vi "readMotorPodConfig.vi"(7 "Input Pod Clustor":T1, 8 "Pod Number":i32, 9 "Refnum in":T2) -> (1 "Pod Output":T1)   [LabVIEW 2014]
uses:
  <vilib>/Utility/config.llb/Config Data RefNum.ctl
  read/readI32.vi
  read/readDoubleKey.vi
  read/readBooleanKey.vi
  read/readStringKey.vi
  <vilib>/Utility/config.llb/NI_LVConfig.lvlib
panel:
  in  "error in (no error)":errorcluster
  out "Refnum out":T2
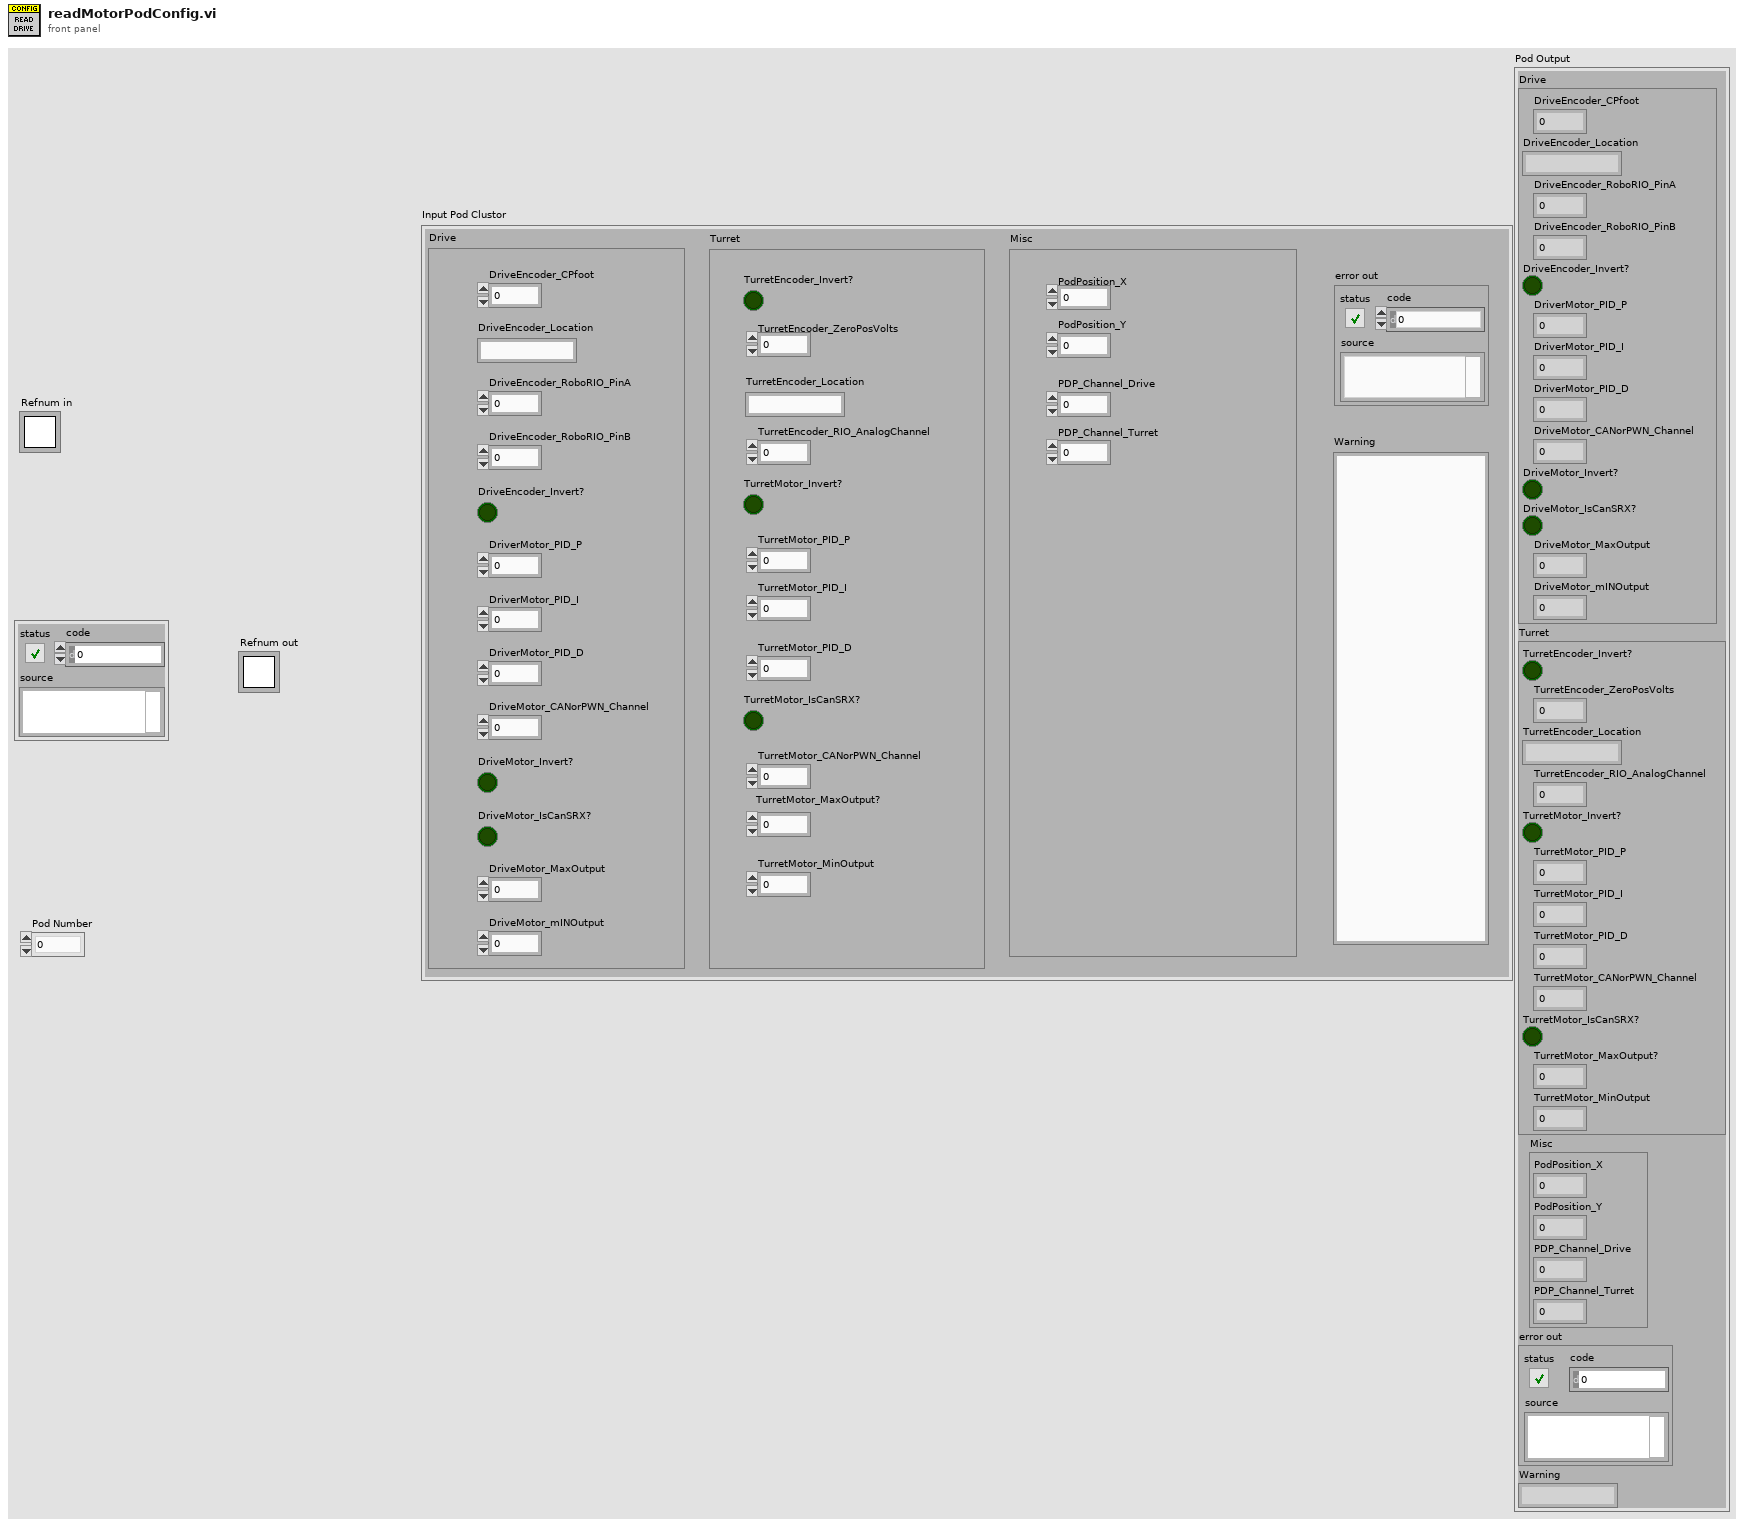
[diagram p1: front panel]
types:
  T1 = cluster{"Drive":cluster{"DriveEncoder_CPfoot":dbl, "DriveEncoder_Location":string, "DriveEncoder_RoboRIO_PinA":i32, "DriveEncoder_RoboRIO_PinB":i32, "DriveEncoder_Invert?":bool, "DriverMotor_PID_P":dbl, "DriverMotor_PID_I":dbl, "DriverMotor_PID_D":dbl, "DriveMotor_CANorPWN_Channel":i32, "DriveMotor_Invert?":bool, "DriveMotor_IsCanSRX?":bool, "DriveMotor_MaxOutput":dbl, "DriveMotor_mINOutput":dbl}, "Turret":cluster{"TurretEncoder_Invert?":bool, "TurretEncoder_ZeroPosVolts":dbl, "TurretEncoder_Location":string, "TurretEncoder_RIO_AnalogChannel":dbl, "TurretMotor_Invert?":bool, "TurretMotor_PID_P":dbl, "TurretMotor_PID_I":dbl, "TurretMotor_PID_D":dbl, "TurretMotor_CANorPWN_Channel":dbl, "TurretMotor_IsCanSRX?":bool, "TurretMotor_MaxOutput?":dbl, "TurretMotor_MinOutput":dbl}, "Misc":cluster{"PodPosition_X":dbl, "PodPosition_Y":dbl, "PDP_Channel_Drive":i32, "PDP_Channel_Turret":i32}, "error out":errorcluster, "Warning":string}
  T2 = typedef "NI_LVConfig.lvlib/Config Data RefNum.ctl" = refnum<k1>
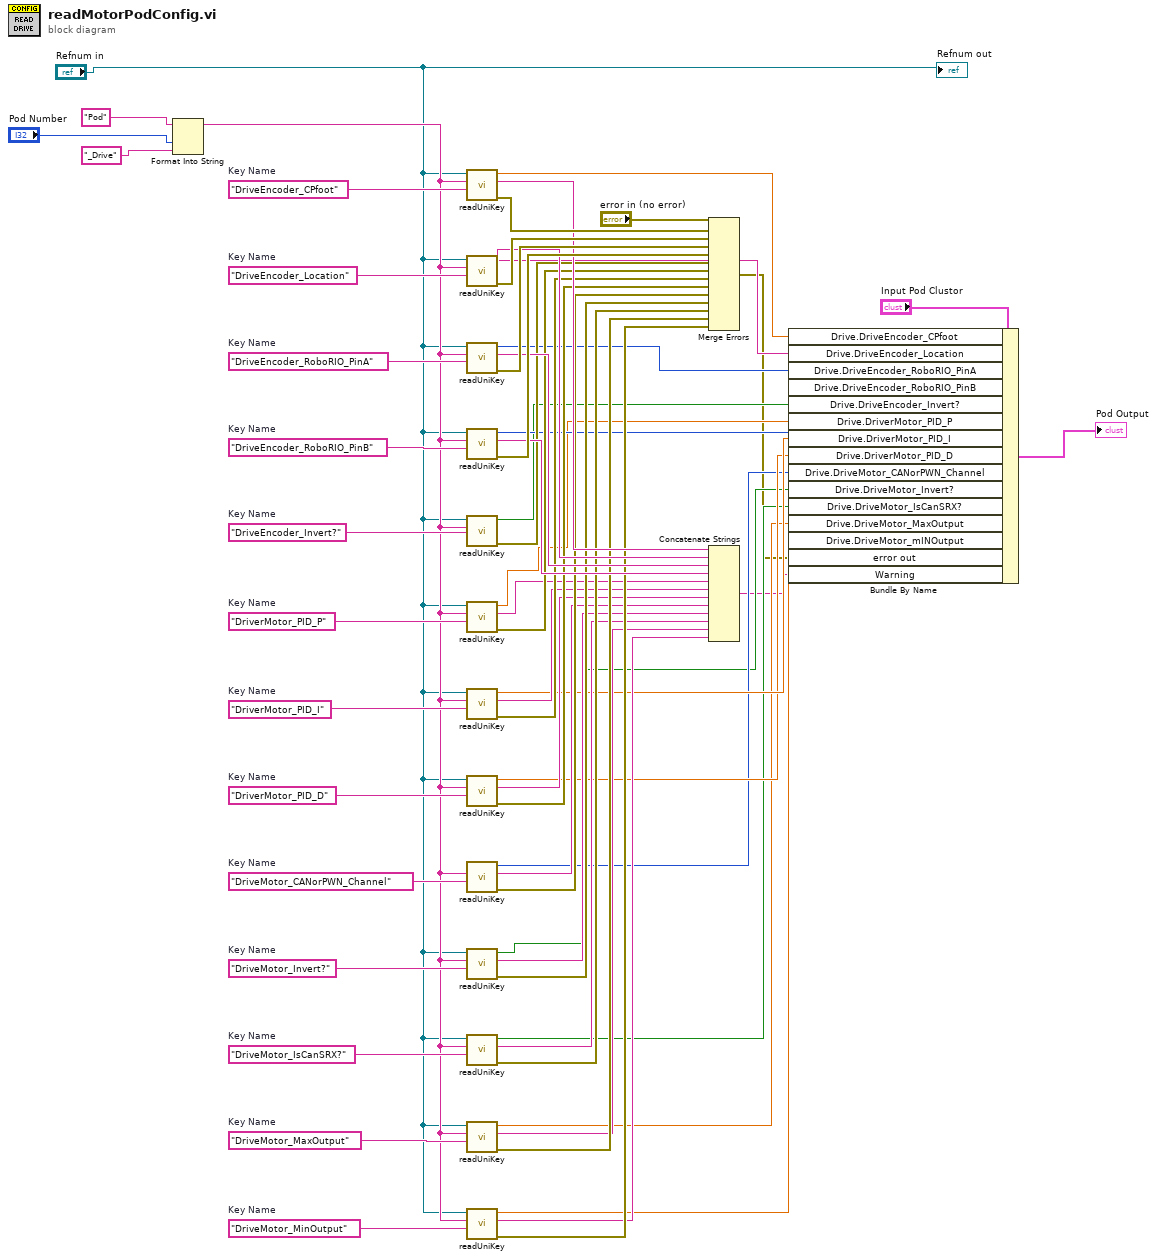
[diagram p0: block diagram]
diagram:
  w38 = "DriveMotor_MinOutput"  # Key Name
  w40 = "DriveMotor_MaxOutput"  # Key Name
  w39 = "DriveMotor_IsCanSRX?"  # Key Name
  w41 = "DriveMotor_Invert?"  # Key Name
  w42 = "DriveMotor_CANorPWN_Channel"  # Key Name
  w45 = "DriverMotor_PID_D"  # Key Name
  w46 = "DriverMotor_PID_I"  # Key Name
  w44 = "DriverMotor_PID_P"  # Key Name
  w43 = "DriveEncoder_Invert?"  # Key Name
  w59 = "DriveEncoder_RoboRIO_PinB"  # Key Name
  w58 = "DriveEncoder_RoboRIO_PinA"  # Key Name
  w60 = "DriveEncoder_Location"  # Key Name
  w61 = "DriveEncoder_CPfoot"  # Key Name
  n1 = Format Into String(initial string="Pod", "Pod Number", "_Drive") -> (resulting string=w37:string)  [unwired: 2 in, 1 out]
  n2 = call-poly "readUniKey.vi"("Refnum in"="Refnum in", "Section"=w37, "Key Name"=w61) -> ("value"=w15:dbl, "Warning"=w53:string, "error out"=w57:errorcluster)  [unwired: 5 in]
  n3 = call-poly "readUniKey.vi"("Refnum in"="Refnum in", "Section"=w37, "Key Name"=w60) -> ("value"=w14:string, "Warning"=w52:string, "error out"=w56:errorcluster)  [unwired: 5 in]
  n4 = call-poly "readUniKey.vi"("Refnum in"="Refnum in", "Section"=w37, "Key Name"=w58) -> ("value"=w13:i32, "Warning"=w51:string, "error out"=w55:errorcluster)  [unwired: 5 in]
  n5 = call-poly "readUniKey.vi"("Refnum in"="Refnum in", "Section"=w37, "Key Name"=w59) -> ("value"=w12:i32, "Warning"=w50:string, "error out"=w54:errorcluster)  [unwired: 5 in]
  n6 = call-poly "readUniKey.vi"("Refnum in"="Refnum in", "Section"=w37, "Key Name"=w43) -> ("value"=w11:bool, "error out"=w36:errorcluster)  [unwired: 5 in, 1 out]
  n7 = call-poly "readUniKey.vi"("Refnum in"="Refnum in", "Section"=w37, "Key Name"=w44) -> ("value"=w10:dbl, "Warning"=w27:string, "error out"=w35:errorcluster)  [unwired: 5 in]
  n8 = call-poly "readUniKey.vi"("Refnum in"="Refnum in", "Section"=w37, "Key Name"=w46) -> ("value"=w9:dbl, "Warning"=w26:string, "error out"=w34:errorcluster)  [unwired: 5 in]
  n9 = call-poly "readUniKey.vi"("Refnum in"="Refnum in", "Section"=w37, "Key Name"=w45) -> ("value"=w8:dbl, "Warning"=w25:string, "error out"=w33:errorcluster)  [unwired: 5 in]
  n10 = call-poly "readUniKey.vi"("Section"=w37, "Key Name"=w42) -> ("value"=w7:i32, "Warning"=w24:string, "error out"=w32:errorcluster)  [unwired: 6 in]
  n11 = call-poly "readUniKey.vi"("Refnum in"="Refnum in", "Section"=w37, "Key Name"=w41) -> ("value"=w6:bool, "Warning"=w23:string, "error out"=w31:errorcluster)  [unwired: 5 in]
  n12 = call-poly "readUniKey.vi"("Refnum in"="Refnum in", "Section"=w37, "Key Name"=w39) -> ("value"=w5:bool, "Warning"=w22:string, "error out"=w30:errorcluster)  [unwired: 5 in]
  n13 = call-poly "readUniKey.vi"("Refnum in"="Refnum in", "Section"=w37, "Key Name"=w40) -> ("value"=w4:dbl, "Warning"=w21:string, "error out"=w29:errorcluster)  [unwired: 5 in]
  n14 = call-poly "readUniKey.vi"("Refnum in"="Refnum in", "Section"=w37, "Key Name"=w38) -> ("value"=w3:dbl, "Warning"=w20:string, "error out"=w28:errorcluster)  [unwired: 5 in]
  n15 = Merge Errors "Merge Errors"("error in (no error)", w57, w56, w55, w54, w36, w35, w34, w33, w32, w31, w30, w29, w28) -> (w2:errorcluster)
  n16 = Concatenate Strings ("Concatenate Warnings")(w53, w52, w51, w50, w27, w26, w25, w24, w23, w22, w21, w20) -> (w1:string)
  n17 = Bundle By Name(cluster="Input Pod Clustor", "Drive.DriveEncoder_CPfoot"=w15, "Drive.DriveEncoder_Location"=w14, "Drive.DriveEncoder_RoboRIO_PinA"=w13, "Drive.DriveEncoder_RoboRIO_PinB"=w12, "Drive.DriveEncoder_Invert?"=w11, "Drive.DriverMotor_PID_P"=w10, "Drive.DriverMotor_PID_I"=w9, "Drive.DriverMotor_PID_D"=w8, "Drive.DriveMotor_CANorPWN_Channel"=w7, "Drive.DriveMotor_Invert?"=w6, "Drive.DriveMotor_IsCanSRX?"=w5, "Drive.DriveMotor_MaxOutput"=w4, "Drive.DriveMotor_mINOutput"=w3, "error out"=w2, "Warning"=w1) -> (→"Pod Output":T1)
  "Refnum out" <- "Refnum in"
